vi "runtest execute.vi"(6 "User/Station":T8, 7 "POST (empty)":T1, 8 "error in (no error)":errorcluster, 9 "Fields / Results":T6, 10 "Test Sequence ID":string, 11 "Connection Refnum":T7) -> (0 "error out":errorcluster, 1 "Updated Fields / Results":T6, 2 "dup Test Sequence ID":string, 3 "Connection Refnum":T7, 4 "Next Item?":bool, 5 "POST out":T1)   [LabVIEW 2011]
uses:
  runtest User - Station.ctl
  server/database/Stations/Instruments/Instrument Record.ctl
  server/database/Stations/Step Associations/Step Association Record.ctl
  Addons/internet/utils/keyedarr.llb/Keyed Array.ctl
  SI.LIB/ODBC/SQL Controls/Connection Refnum.ctl
  server/database/Fields/Field Record.ctl
  server/database/Fields/Field DataTypes.ctl
  server/database/Fields/Field NextItem.ctl
  tests/Test Output.ctl
  server/database/Fields/Field System Fields.ctl
  Addons/internet/utils/strutil.llb/Case Matching.ctl
  tests/Get Instruments Required From Test Step.vi
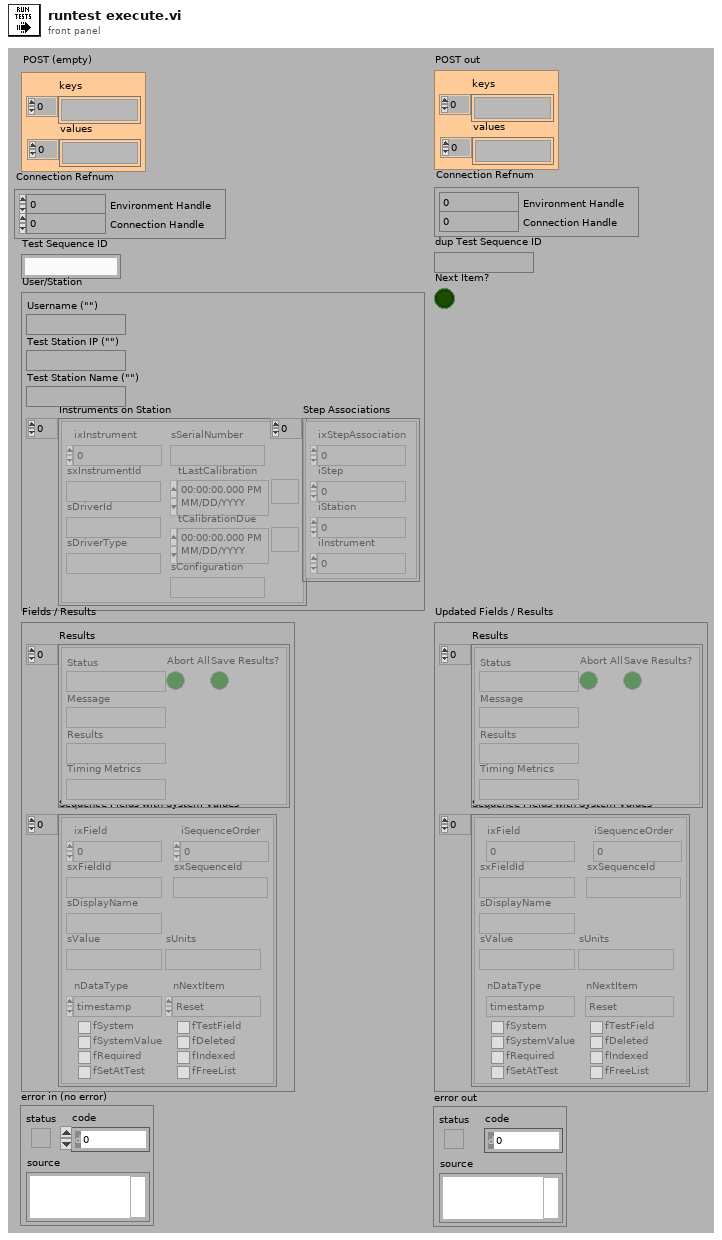
[diagram p1: front panel]
types:
  T1 = typedef "Keyed Array.ctl" = cluster{"keys":string[], "values":string[]}
  T2 = typedef "Field Record.ctl" = cluster{"ixField":i32, "iSequenceOrder":i32, "sxFieldId":string, "sxSequenceId":string, "sDisplayName":string, "sValue":string, "sUnits":string, "nDataType":T3, "nNextItem":T4, "fSystem":bool, "fSystemValue":bool, "fRequired":bool, "fSetAtTest":bool, "fTestField":bool, "fDeleted":bool, "fIndexed":bool, "fFreeList":bool}
  T3 = typedef "Field DataTypes.ctl" = enum32{"text", "numeric", "list", "timestamp", "boolean"}
  T4 = typedef "Field NextItem.ctl" = enum32{"Reset", "Retain", "Auto-Increment"}
  T5 = typedef "Test Output.ctl" = cluster{"Status":string, "Message":string, "Results":string, "Abort All":bool, "Save Results?":bool, "Timing Metrics":string}
  T6 = cluster{"Sequence Fields with System Values":T2[], "Results":T5[]}
  T7 = typedef "Connection Refnum.ctl" = cluster{"Environment Handle":i32, "Connection Handle":i32}
  T8 = typedef "runtest User - Station.ctl" = cluster{"Username (\"\")":string, "Test Station IP (\"\")":string, "Test Station Name (\"\")":string, "Instruments on Station":T9[], "Step Associations":T10[]}
  T9 = typedef "Instrument Record.ctl" = cluster{"ixInstrument":i32, "sxInstrumentId":string, "sDriverId":string, "sDriverType":string, "sSerialNumber":string, "tLastCalibration":timestamp, "tCalibrationDue":timestamp, "sConfiguration":string}
  T10 = typedef "Step Association Record.ctl" = cluster{"ixStepAssociation":i32, "iStep":i32, "iStation":i32, "iInstrument":i32}
  T11 = typedef "Field System Fields.ctl" = enum32{"Company", "End_Timestamp", "Model_Number", "Operator", "Serial_Number", "Start_Timestamp", "Step_Number", "Step_Tag", "Test_Run", "Test_Sequence", "Test_Station", "Test_Station_Name", "Test_Status", "Test_Type", "Test_Version", "Spartan_Version_Created", "Spartan_Version_Current"}
  T12 = typedef "Sequence Record.ctl" = cluster{"ixSequence":i32, "sxSequenceId":string, "sDescription":string, "sCreator":string, "tCreationDate":timestamp, "sModifier":string, "tModifiedDate":timestamp, "fApproved":bool, "fSpartanSetsSN":bool, "fOverwriteData":bool, "fStopOnFail":bool, "fDisableQuickMode":bool, "fPartialExecution":bool, "fAutoNextItem":bool, "fDoNotPrintOnFail":bool}
  T13 = typedef "Step Record.ctl" = cluster{"ixStep":i32, "sxSequenceId":string, "sxTestId":string, "iIndex":i32, "iRepeat":i32, "iQuickMode":i32, "sTag":string, "sDatasheetsCSV":string, "bConfiguration":string}
  T14 = typedef "Case Matching.ctl" = enum16{"a != A", "a == A", "system"}
  T15 = typedef "Test Execution Settings.ctl" = cluster{"Quick Mode (T)":bool, "Seq Count":i32, "Step Info":string, "Instruments on Station":T9[], "LANGUAGE":string, "Files Found?":bool, "Step Number":i32}
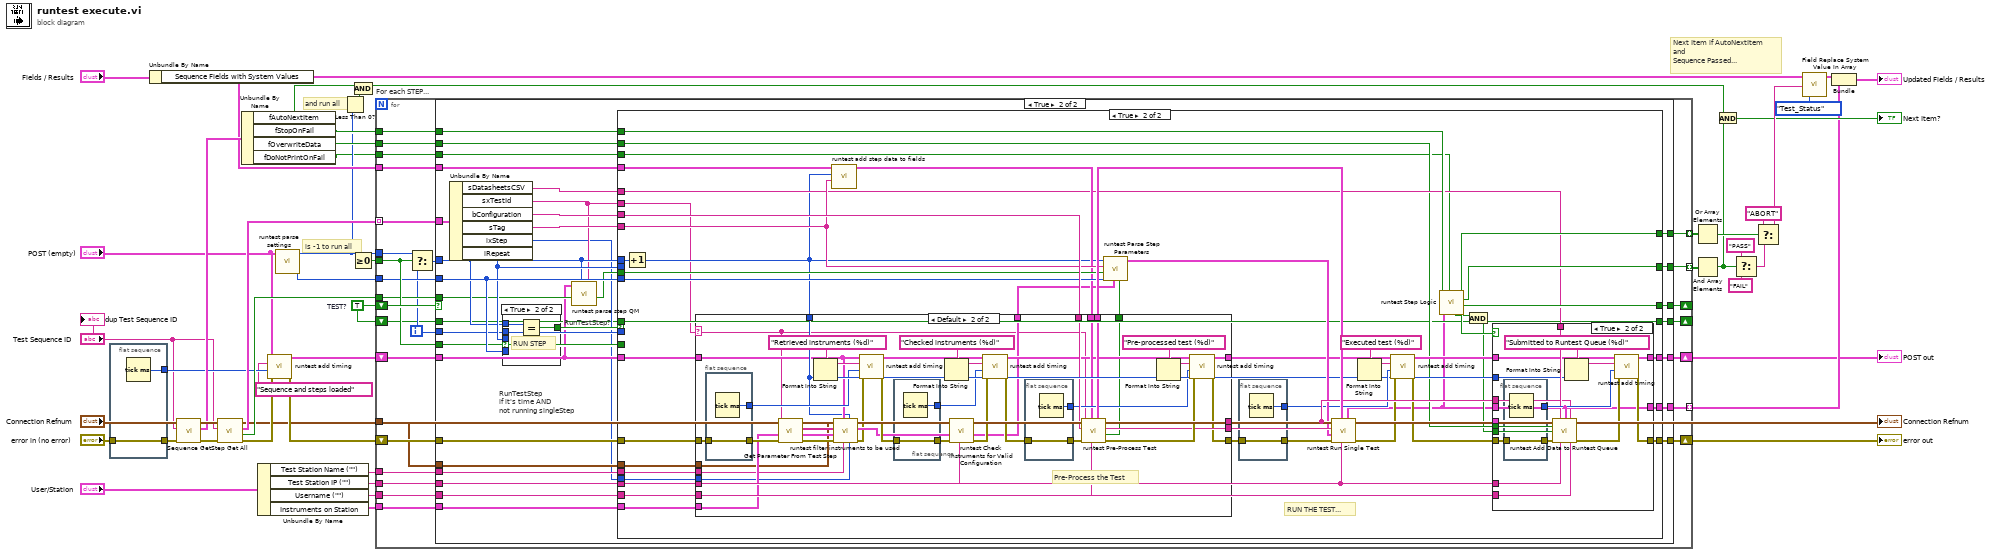
[diagram p0: block diagram]
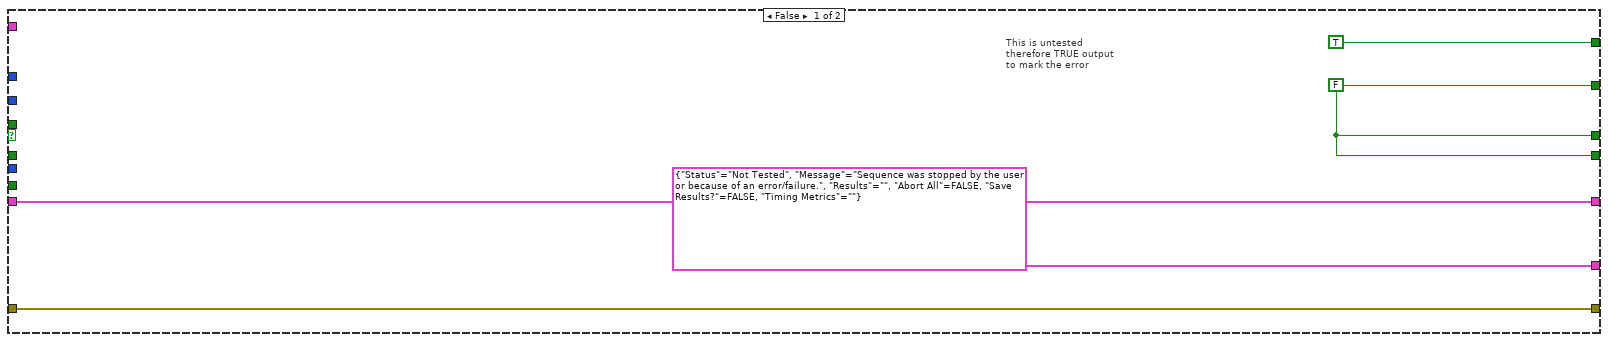
[diagram p2: hidden frame]
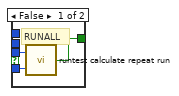
[diagram p3: hidden frame]
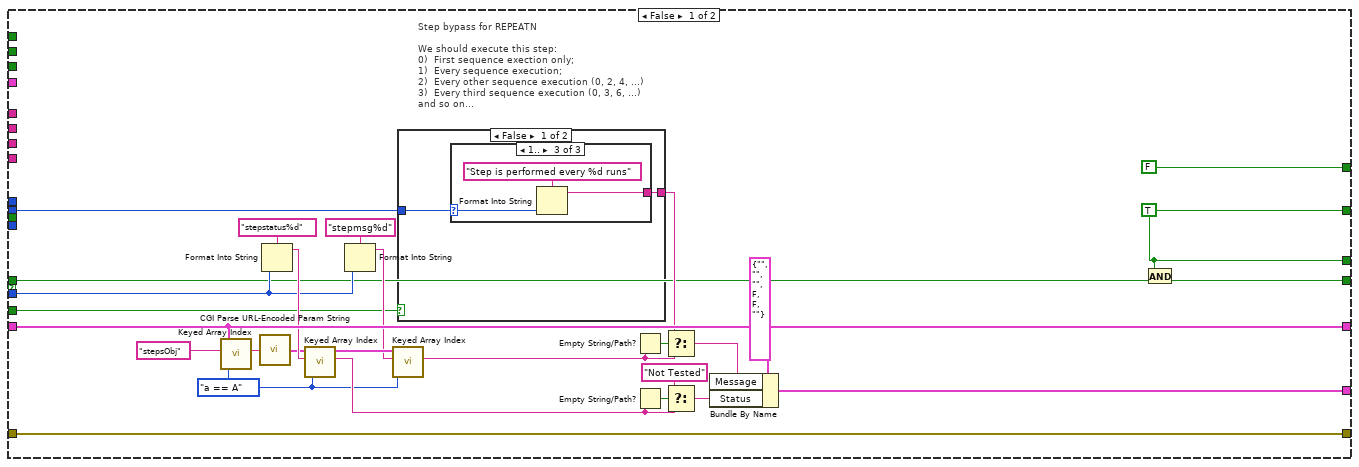
[diagram p4: hidden frame]
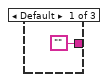
[diagram p5: hidden frame]
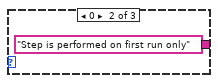
[diagram p6: hidden frame]
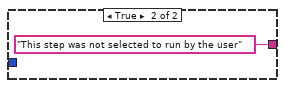
[diagram p7: hidden frame]
diagram:
  w1 = TRUE  # TEST?
  # "is -1 to run all"
  # "and run all"
  # "Next Item if AutoNextItem\nand\nSequence Passed..."
  n1 = flat-sequence {
    tunnel: "error in (no error)" -> [w51]
    tunnel: [w51] -> w21
    tunnel: [w50] -> w20
    frame #0 {
      n2 = Tick Count (ms)() -> (millisecond timer value=w50:u32)
    }
  }
  n3 = Unbundle By Name("Fields / Results") -> ("Sequence Fields with System Values"=w9:T2[])
  n4 = call "Sequence Get.vi"("error in (no error)"=w21, "sxSequenceId (\"\")"="Test Sequence ID", "Connection Refnum"="Connection Refnum") -> ("error out"=w37:errorcluster, "Sequence Record"=w34:T12, "Connection Refnum"=w38:T7)  [unwired: 6 out]
  n5 = call "Step Get All.vi"("error in (no error)"=w37, "sxSequenceId"="Test Sequence ID", "Connection Refnum"=w38) -> ("error out"=w16:errorcluster, "Any Quickmode Allowed?"=w28:bool, "Sequence Steps"=w35:T13[], "Connection Refnum"=w4:T7)  [unwired: 1 in, 4 out]
  "Connection Refnum" <- w4
  n6 = Unbundle By Name(w34) -> ("fAutoNextItem"=w7:bool, "fStopOnFail"=w33:bool, "fOverwriteData"=w32:bool, "fDoNotPrintOnFail"=w2:bool)
  n7 = Unbundle By Name("User/Station") -> ("Test Station Name (\"\")"=w3:string, "Test Station IP (\"\")"=w11:string, "Username (\"\")"=w10:string, "Instruments on Station"=w27:T9[])
  n8 = call "runtest add timing.vi"("error in (no error)"=w16, "Start Tick, ms (0)"=w20, "Function (\"\")"="Sequence and steps loaded" ("Where?"), "POST (empty)"="POST (empty)") -> ("error out"=w15:errorcluster, "POST out"=w17:T1)  [unwired: 6 out]
  n9 = call "runtest parse settings.vi"("POST (empty)"="POST (empty)") -> ("SeqCount"=w30:i32, "Run Step"=w6:i32)  [unwired: 1 in, 8 out]
  n10 = Less Than 0?(x=w6) -> (x < 0?=w5:bool)
  n11 = Greater Or Equal To 0?(x=w6) -> (x >= 0?=w40:bool)
  n12 = And(x=w7, y=w5) -> (x .and. y?=w8:bool)
  n13 = for "For each STEP..." {
    shift-right: [w77] -> w14
    shift-left: w15 -> [w78]
    tunnel: w27 -> [w76]
    tunnel: w9 -> [w75]
    tunnel: w6 -> [w74]
    tunnel: w35 -> [w73] mode=indexing
    tunnel: w40 -> [w68]
    tunnel: [w71] -> w49 mode=indexing
    shift-right: [w69] -> _
    shift-left: w1 -> [w70]
    tunnel: w30 -> [w67]
    tunnel: w11 -> [w66]
    tunnel: w10 -> [w65]
    tunnel: [w64] -> w45 mode=indexing
    tunnel: w28 -> [w63]
    tunnel: [w62] -> w24 mode=indexing
    tunnel: w33 -> [w61]
    tunnel: w32 -> [w60]
    shift-right: [w58] -> w13
    shift-left: w17 -> [w59]
    tunnel: w4 -> [w56]
    tunnel: w3 -> [w55]
    tunnel: w2 -> [w54]
    shift-right: [w53] -> _
    shift-left: w1 -> [w52]
    i -> [w57]
    n14 = Select(t=w74, s=w68, f=w57) -> (s? t:f=w72:i32)
    n15 = case shown="True" w70 {
      tunnel: w78 -> [w82 w93]
      tunnel: [w82 w116] -> w77
      tunnel: w76 -> [_ w115]
      tunnel: w75 -> [_ w114]
      tunnel: w73 -> [_ w113]
      tunnel: w72 -> [_ w98]
      tunnel: [w79 w108] -> w71
      tunnel: w60 -> [_ w111]
      tunnel: w61 -> [_ w110]
      tunnel: [w79 w109] -> w69
      tunnel: w68 -> [_ w100]
      tunnel: w67 -> [_ w104]
      tunnel: w66 -> [_ w106]
      tunnel: w65 -> [_ w105]
      tunnel: [TRUE w103] -> w64
      tunnel: w63 -> [_ w97]
      tunnel: [T5 {"Status"="Not Tested", "Message"="Sequence was stopped by the user or because of an error/failure.", "Results"="", "Abort All"=FALSE, "Save Results?"=FALSE, "Timing Metrics"=""} ("Test Output") w101] -> w62
      tunnel: w57 -> [_ w91]
      tunnel: w59 -> [w80 w89]
      tunnel: [w80 w94] -> w58
      tunnel: w56 -> [_ w90]
      tunnel: w55 -> [_ w88]
      tunnel: w54 -> [_ w86]
      tunnel: [w79 w85] -> w53
      tunnel: w52 -> [_ w84]
      frame False {
        w79 = FALSE
        # "This is untested\ntherefore TRUE output\nto mark the error"
      }
      frame True {
        # "RunTestStep?"
        # "RunTestStep\nif it's time AND\nnot running singleStep"
        n16 = Unbundle By Name(w113) -> ("sDatasheetsCSV"=w92:string, "sxTestId"=w95:string, "bConfiguration"=w112:string, "sTag"=w99:string, "ixStep"=w87:i32, "iRepeat"=w102:i32)
        n17 = case shown="True" w100 {
          tunnel: [w117 w121] -> w107
          tunnel: w102 -> [w119 _]
          tunnel: w104 -> [w118 _]
          tunnel: w98 -> [_ w122]
          tunnel: w91 -> [_ w120]
          frame False {
            # "RUNALL"
            n18 = call "runtest calculate repeat run.vi"("SeqCount"=w118, "Repeat N"=w119) -> ("RUN?"=w117:bool)
          }
          frame True {
            # "RUN STEP"
            n19 = Equal?(x=w122, y=w120) -> (x = y?=w121:bool)
          }
        }
        n20 = call "runtest parse step QM.vi"("Step Test ID"=w95, "Step Number"=w98, "Sequence QM allowed?"=w97, "POST (empty)"=w89) -> ("Quickmode?"=w96:bool)  [unwired: 7 out]
        n21 = case shown="True" w107 {
          tunnel: [w148 w203] -> w116
          tunnel: w93 -> [w148 w202]
          tunnel: w115 -> [_ w194]
          tunnel: w114 -> [_ w187]
          tunnel: w95 -> [_ w160]
          tunnel: w112 -> [_ w205]
          tunnel: w98 -> [_ w206]
          tunnel: w111 -> [_ w165]
          tunnel: w110 -> [_ w198]
          tunnel: [w123 w196] -> w109
          tunnel: [w123 w197] -> w108
          tunnel: w106 -> [_ w172]
          tunnel: w105 -> [_ w204]
          tunnel: w99 -> [_ w191]
          tunnel: w104 -> [_ w193]
          tunnel: [FALSE w199] -> w103
          tunnel: w102 -> [w149 _]
          tunnel: w96 -> [_ w192]
          tunnel: [w146 w200] -> w101
          tunnel: w100 -> [w127 _]
          tunnel: w89 -> [w145 w170]
          tunnel: [w145 w175] -> w94
          tunnel: w92 -> [_ w174]
          tunnel: w91 -> [w126 _]
          tunnel: w90 -> [_ w166]
          tunnel: w88 -> [_ w168]
          tunnel: w87 -> [_ w167]
          tunnel: w86 -> [_ w164]
          tunnel: [w125 w162] -> w85
          tunnel: w84 -> [w124 w161]
          frame False {
            w129 = Case_Matching."a == A" ("case matching (sensitive)")
            w123 = TRUE
            # "Step bypass for REPEATN\n\nWe should execute this step:\n0)  First sequence exection only;\n1)  Every sequence execution;\n2)  Every other sequence execution (0, 2, 4, ...)\n3)  Every third sequence execution (0, 3, 6, ...)\nand so on..."
            n22 = call "Keyed Array Index.vi"("case matching (sensitive)"=w129, "key"="stepsObj", "array in"=w145) -> ("value"=w143:string)  [unwired: 1 in, 3 out]
            n23 = call "CGI Parse URL-Encoded Param String.vi"("url-encoded param string"=w143) -> ("params"=w128:T1)
            n24 = Format Into String(format string="stepstatus%d" ("key"), w126) -> (resulting string=w138:string)  [unwired: 2 in, 1 out]
            n25 = call "Keyed Array Index.vi"("case matching (sensitive)"=w129, "key"=w138, "array in"=w128) -> ("value"=w132:string, "duplicate array"=w140:T1)  [unwired: 1 in, 2 out]
            n26 = Format Into String(format string="stepmsg%d" ("key"), w126) -> (resulting string=w139:string)  [unwired: 2 in, 1 out]
            n27 = call "Keyed Array Index.vi"("case matching (sensitive)"=w129, "key"=w139, "array in"=w140) -> ("value"=w136:string)  [unwired: 1 in, 3 out]
            n28 = case shown="False" w127 {
              tunnel: w149 -> [w152 _]
              tunnel: [w151 "This step was not selected to run by the user" ("Status")] -> w134
              frame False {
                n29 = case shown="1.." w152 {
                  selector: w152 -> [_ _ w155]
                  tunnel: ["" "Step is performed on first run only" ("Status") w157] -> w151
                  frame Default {
                  }
                  frame 0 {
                  }
                  frame 1.. {
                    n30 = Format Into String(format string="Step is performed every %d runs" ("Status"), w155) -> (resulting string=w157:string)  [unwired: 2 in, 1 out]
                  }
                }
              }
              frame True {
              }
            }
            n31 = Empty String/Path?(string/path=w136) -> (empty?=w137:bool)
            n32 = Empty String/Path?(string/path=w132) -> (empty?=w133:bool)
            n33 = Select(t=w134, s=w137, f=w136) -> (s? t:f=w135:string)
            n34 = Select(t="Not Tested", s=w133, f=w132) -> (s? t:f=w131:string)
            n35 = Bundle By Name(cluster=T5 {"Status"="", "Message"="", "Results"="", "Abort All"=FALSE, "Save Results?"=FALSE, "Timing Metrics"=""} ("Test Output"), "Message"=w135, "Status"=w131) -> (w146:T5)
            n36 = And(x=w123, y=w124) -> (x .and. y?=w125:bool)
          }
          frame True {
            # "RUN THE TEST..."
            n37 = Increment(x=w206) -> (x+1=w169:i32)
            n38 = call "runtest add step data to fields.vi"("Step Tag"=w191, "Step Number"=w169, "Fields Array"=w187) -> ("Fields Array"=w186:T2[])  [unwired: 8 out]
            n39 = case shown="Default" w160 {
              selector: w160 -> [w207 w212]
              tunnel: w205 -> [w208 w254]
              tunnel: w204 -> [_ w253]
              tunnel: w202 -> [w209 w251]
              tunnel: [w211 w247] -> w201
              tunnel: w194 -> [_ w245]
              tunnel: [w207 w241] -> w190
              tunnel: [w208 w239] -> w188
              tunnel: w186 -> [w211 w238]
              tunnel: [w209 w237] -> w184
              tunnel: [w210 w236] -> w177
              tunnel: [_ w226] -> w173
              tunnel: w172 -> [_ w225]
              tunnel: [_ w224] -> w171
              tunnel: w170 -> [w210 w223]
              tunnel: w169 -> [_ w217]
              tunnel: w168 -> [_ w216]
              tunnel: w167 -> [_ w215]
              tunnel: w166 -> [_ w214]
              frame "Prompt", "Prompted Inputs" {
              }
              frame Default {
                # "Pre-Process the Test"
                n40 = flat-sequence {
                  tunnel: [w260] -> w252
                  tunnel: w251 -> [w259]
                  tunnel: [w259] -> w250
                  frame #0 {
                    n41 = Tick Count (ms)() -> (millisecond timer value=w260:u32)
                  }
                }
                n42 = call-poly "Get Parameter From Test Step.vi"("error in (no error)"=w250, "Instruments on Station"=w245, "Test_ID (\"\")"=w212) -> ("error out"=w221:errorcluster, "Required Instruments"=w219:T9[], "Instrument Types"=w218:string[])  [unwired: 6 out]
                n43 = Format Into String(format string="Retrieved instruments (%d)", w217) -> (resulting string=w248:string)  [unwired: 2 in, 1 out]
                n44 = call "runtest filter instruments to be used.vi"("ixStep"=w215, "Step Number"=w217, "sxStationId"=w216, "POST (empty)"=w223, "error in (no error)"=w221, "Instruments In"=w219, "Instrument Types"=w218, "Connection Refnum"=w214) -> ("error out"=w220:errorcluster, "Instruments Out"=w222:T9[], "Connection Refnum"=w213:T7)  [unwired: 1 in]
                n45 = call "runtest add timing.vi"("error in (no error)"=w220, "Start Tick, ms (0)"=w252, "Function (\"\")"=w248, "POST (empty)"=w223) -> ("error out"=w234:errorcluster, "POST out"=w231:T1)  [unwired: 6 out]
                n46 = flat-sequence {
                  tunnel: [w256] -> w235
                  tunnel: w234 -> [w255]
                  tunnel: [w255] -> w228
                  frame #0 {
                    n47 = Tick Count (ms)() -> (millisecond timer value=w256:u32)
                  }
                }
                n48 = Format Into String(format string="Checked instruments (%d)", w217) -> (resulting string=w232:string)  [unwired: 2 in, 1 out]
                n49 = call "runtest Check Instruments for Valid Configuration.vi"("TestStation IP (\"\")"=w225, "error in (no error)"=w228, "Required Instruments In"=w222, "Connection Refnum"=w213) -> ("error out"=w227:errorcluster, "Required Instruments Out"=w226:T9[])  [unwired: 6 out]
                n50 = call "runtest add timing.vi"("error in (no error)"=w227, "Start Tick, ms (0)"=w235, "Function (\"\")"=w232, "POST (empty)"=w231) -> ("error out"=w229:errorcluster, "POST out"=w230:T1)  [unwired: 6 out]
                n51 = flat-sequence {
                  tunnel: [w258] -> w240
                  tunnel: w229 -> [w257]
                  tunnel: [w257] -> w246
                  frame #0 {
                    n52 = Tick Count (ms)() -> (millisecond timer value=w258:u32)
                  }
                }
                n53 = call "runtest Pre-Process Test.vi"("Username (\"\")"=w253, "Fields In"=w238, "error in (no error)"=w246, "Test Configuration (\"\")"=w254, "Test_ID (\"\")"=w212) -> ("error out"=w242:errorcluster, "Files Found?"=w224:bool, "New Test Configuration"=w239:string, "Test_ID Out"=w241:string, "Fields Out"=w247:T2[])  [unwired: 2 out]
                n54 = Format Into String(format string="Pre-processed test (%d)", w217) -> (resulting string=w244:string)  [unwired: 2 in, 1 out]
                n55 = call "runtest add timing.vi"("error in (no error)"=w242, "Start Tick, ms (0)"=w240, "Function (\"\")"=w244, "POST (empty)"=w230) -> ("error out"=w237:errorcluster, "POST out"=w236:T1)  [unwired: 6 out]
              }
            }
            n56 = call "runtest Parse Step Parameters.vi"("Files Found?"=w171, "Instruments on Station"=w173, "Sequence Count (0)"=w193, "Quickmode? (f)"=w192, "Step Tab (\"\")"=w191, "Step Number (0)"=w169) -> ("Step parameters"=w185:T15)  [unwired: 5 out]
            n57 = flat-sequence {
              tunnel: [w262] -> w180
              tunnel: w184 -> [w261]
              tunnel: [w261] -> w183
              frame #0 {
                n58 = Tick Count (ms)() -> (millisecond timer value=w262:u32)
              }
            }
            n59 = call "runtest Run Single Test.vi"("TestStation IP (\"\")"=w172, "Fields In"=w201, "error in (no error)"=w183, "Test Execution Settings"=w185, "Test Configuration (\"\")"=w188, "Test_ID (\"\")"=w190) -> ("error out"=w179:errorcluster, "Fields Out"=w189:T2[], "Test Output"=w159:T5)  [unwired: 1 in, 2 out]
            n60 = Format Into String(format string="Executed test (%d)", w169) -> (resulting string=w181:string)  [unwired: 2 in, 1 out]
            n61 = call "runtest add timing.vi"("error in (no error)"=w179, "Start Tick, ms (0)"=w180, "Function (\"\")"=w181, "POST (empty)"=w177) -> ("error out"=w178:errorcluster, "POST out"=w176:T1)  [unwired: 6 out]
            n62 = call "runtest Step Logic.vi"("Do Not Print On Fail? (f)"=w164, "Step Results (empty)"=w159, "Stop on First Fail? (f)"=w198) -> ("Save Data?"=w195:bool, "Continue Testing?"=w196:bool, "Not Aborted OR Error OR Fail?"=w197:bool, "Not Pass OR Fail?"=w199:bool, "Print?"=w163:bool)  [unwired: 4 in]
            n63 = And(x=w163, y=w161) -> (x .and. y?=w162:bool)
            n64 = case shown="True" w195 {
              tunnel: [w265 w276] -> w203
              tunnel: w204 -> [_ w283]
              tunnel: w178 -> [w265 w271]
              tunnel: w172 -> [_ w282]
              tunnel: w159 -> [w264 w270]
              tunnel: w190 -> [_ w269]
              tunnel: [w264 w270] -> w200
              tunnel: w189 -> [_ w268]
              tunnel: w176 -> [w263 w272]
              tunnel: [w263 w278] -> w175
              tunnel: w169 -> [_ w273]
              tunnel: w174 -> [_ w274]
              tunnel: w165 -> [_ w267]
              tunnel: w162 -> [_ w266]
              frame False {
              }
              frame True {
                n65 = flat-sequence {
                  tunnel: [w285] -> w275
                  tunnel: w271 -> [w284]
                  tunnel: [w284] -> w281
                  frame #0 {
                    n66 = Tick Count (ms)() -> (millisecond timer value=w285:u32)
                  }
                }
                n67 = call "runtest Add Data to Runtest Queue.vi"("Fields"=w268, "sDatasheetsCSV (\"\")"=w274, "Test Output"=w270, "sTestId"=w269, "Overwrite Existing?"=w267, "Print?"=w266, "error in (no error)"=w281, "Test Station IP (\"\")"=w282, "sxUsername (\"\")"=w283) -> ("error out"=w277:errorcluster)  [unwired: 6 in]
                n68 = Format Into String(format string="Submitted to Runtest Queue (%d)", w273) -> (resulting string=w279:string)  [unwired: 2 in, 1 out]
                n69 = call "runtest add timing.vi"("error in (no error)"=w277, "Start Tick, ms (0)"=w275, "Function (\"\")"=w279, "POST (empty)"=w272) -> ("error out"=w276:errorcluster, "POST out"=w278:T1)  [unwired: 6 out]
              }
            }
          }
        }
      }
    }
  }
  "error out" <- w14
  "POST out" <- w13
  n70 = Or Array Elements(Boolean array=w45) -> (logical OR=w44:bool)
  n71 = And Array Elements(Boolean array=w49) -> (logical AND=w31:bool)
  n72 = And(x=w8, y=w31) -> (x .and. y?=→"Next Item?":bool)
  n73 = Select(t="PASS", s=w31, f="FAIL") -> (s? t:f=w42:string)
  n74 = Select(t="ABORT", s=w44, f=w42) -> (s? t:f=w41:string)
  n75 = call "Field Replace System Value In Array.vi"("System Field to Replace (Serial Number)"=Field_System_Fields."Test_Status", "Field Value Replacement Data (\"\")"=w41, "Fields Array In"=w9) -> ("Fields Array Out"=w25:T2[])  [unwired: 1 in, 1 out]
  n76 = Bundle("Fields Array Out"=w25, w24) -> (→"Updated Fields / Results":cluster{"Fields Array Out":T2[], T5[]})  [unwired: 1 out]
  "dup Test Sequence ID" <- "Test Sequence ID"
